vi "nanocal -- nuclear schottky fit V5.vi"() -> ()   [LabVIEW 2020]
uses:
  filename-pattern.ctl
  show-win- control.ctl
  cursor winow.ctl
  nanocal_data_read_format.ctl
  3-lorentzian-parameters.ctl
  nameformattingitem.ctl
  nanocal_side_selector.ctl
  filename-action.ctl
  nanocal -- gradient descent -- parameters.ctl
  3-lorentzian-heat-response action.ctl
  nanocal-goodness-weighting-strategy.ctl
  <vilib>/Analysis/Matrix/Datatypes/RealMatrix.ctl
  <vilib>/Analysis/Matrix/Datatypes/ComplexMatrix.ctl
  cursor window action.ctl
  cursor action.ctl
  2Dwindow.ctl
  publisher action.ctl
  <vilib>/Utility/miscctls.llb/LVMapReplaceAction.ctl
  mathematica string map action.ctl
  agregator -- action.ctl
  nanocal -- gradient descent -- action.ctl
  array action.ctl
  cursor sate.ctl
  nanocal -- defaut parameter manager action-- V1.ctl
  nanocal -- plotstring file action.ctl
  file -- read-write control.ctl
  array -- freq-voltage transformations action.ctl
  nanocal_raw_file_manage_action_V1.ctl
  KM_file -- read-write control.ctl
  replace cursor action stack.vi
  Q -- range multiplier -- real -- V2.vi
  Q - not nan and gtr than zero - Real.vi
  Q - not nan -- real.vi
  Q -- check range -- i -- real.vi
  array - smart min max.vi
  3-lorentzian-heat-response -- V4.vi/142dd4c5-f9ed-c64b-bc14-a88e3e2c450a.vi
  array -- freq-voltage transformations.vi/05c44075-957c-bc42-b6fa-2799d0bc0485.vi
  tale of three indices.vi
  filter -- window span logic.vi
  linear interp iiii- complex - z-omega - divide.vi
  linear interpolation iiii- complex.vi
  containing bix.vi
  <vilib>/Array/Sort 2D Array - Pop Stack.vi
  <vilib>/Array/Sort 2D Array - Push Stack.vi
  array -- freq-voltage transformations.vi/05c44075-957c-bc42-b6fa-2799d0bc0485.vi/5dd0d2be-718e-c148-b8fa-e083cdba2843.vi
  array -- freq-voltage transformations.vi/05c44075-957c-bc42-b6fa-2799d0bc0485.vi/095795a0-771d-c341-9fed-d90d2e44c51c.vi
  command stack.vi
  tale of three indices -- check state.vi
  Q -- check range -- i -- integer.vi
  linear interp iiii- complex - z-omega.vi
  line -- complex.vi
  Q - not nan -- integer.vi
  <vilib>/Analysis/baseanly.llb/A x B.vi
  <vilib>/Analysis/baseanly.llb/Complex A x B.vi
  <vilib>/Analysis/polynomials.llb/Polynomial Roots.vi
  <vilib>/Analysis/polynomials.llb/Polynomial Roots (DBL).vi
  <vilib>/Analysis/Matrix/Numeric/Conversions/Array To Matrix.vi
  <vilib>/Analysis/Matrix/Numeric/Conversions/Array To Matrix - RA2.vi
  <vilib>/Analysis/baseanly.llb/Inverse Matrix.vi
  <vilib>/Analysis/baseanly.llb/Real Inverse Matrix.vi
  <vilib>/Comparison/Less/Less Functor/Less Functor.lvclass
  <vilib>/Analysis/Matrix/NI_Matrix.lvlib
panel:
  in  "tab 10":enum32{"Page 1"}(tab)
  out "curvature tensor":T3
  in  "update curvature plots":bool
  in  "hist size":i32=300
  out "Plot: curvature":cluster{"Freq out (Hz)":dbl[], dbl[]}[](graph)=[{"Freq out (Hz)"=array[300 elements], array[300 elements]}, {"Freq out (Hz)"=[0.04153243950651924, 0.04180026172835088, 0.04258445003699314, 0.0438342337113713, 0.04546073322883233, 0.047333784316083864, 0.049283479875020374, 0.051110588081317194, 0.05260805187888057, 0.05359172755671921, 0.05393366537480654, 0.05358810212962696, 0.05260128268882461, 0.05110153651352443, 0.049273219665611157, 0.04732342294006821, 0.04545126886787391, 0.04382647076923001, 0.042578970605129884, 0.041797433982199705], [0.13184488900598287, 0.13171129861070444, 0.13163855142156844, 0.1316336653013922, 0.13169711120219474, 0.13182276985071803, 0.1319984960783584, 0.13220724864159986, 0.13242869729069096, 0.13264117301723377, 0.13282378589345417, 0.13295850464763131, 0.1330319812802772, 0.13303691930465214, 0.13297282794297968, 0.13284607301385357, 0.13266921842867932, 0.132459736424517, 0.13223823587146255, 0.13202640560334603]}]
  in  "scale gauge: Plot: curvatures":dbl(slide)=0.003141 min=0.0 max=0.3 step=1e-06 scale=1e-09..1.0 scale format="%#_3p"
  in  "radius factor":dbl(slide)=0.01 scale=0.001..1.0 scale format="%#_2p"
  in  "ellipse factor":dbl(slide)=0.0032728445121842026 scale=0.001..1.0 scale format="%#_2p"
  in  "tab 8":enum32{"main", "energy profile", "internals"}(tab)
  out "|dln G/dln α_i |":dbl(slide)=0.0009321298273703344 scale=1e-09..1.0 scale format="%#_3p"
  out "Goodness":dbl(slide)=0.04084184503494657 scale=0.0001..0.5 scale format="%#_3p"
  in  "sweeper panel":enum32{"main"}(tab)
  out "Plot: circles":cluster{"Freq out (Hz)":dbl[], dbl[]}[](graph)
  in  "scale gauge: Plot: circles":dbl(slide)=149590820.049497 min=0.0 max=0.3 step=1e-06 scale=10000000.0..10000000000.0 scale format="%#_3p"
  in  "cspan":dbl=0.003 format="%#_13g"
  in  "tab 77":enum32{"logarithmic derivatives"}(tab)
  in  "factors":cluster{"scaling":dbl, "what":T4}[](array[cluster])=[{"scaling"=1.0, "what"=enum."ζ"}, {"scaling"=1.0, "what"=enum."τ1"}, {"scaling"=1.0, "what"=enum."τS"}, {"scaling"=1.0, "what"=enum."τN"}, {"scaling"=1.0, "what"=enum."τC"}, {"scaling"=1.0, "what"=enum."κ0"}]
  in  "tab77":enum32{"Page 1"}(tab)
  in  "τC":dbl(slide)=0.0011273373743225924 min=0.0 max=0.3 step=1e-06 scale=0.0001..1.0 scale format="%#_3p"
  in  "τN":dbl(slide)=0.017465668384145063 min=0.0 max=0.3 step=1e-06 scale=1e-06..1.0 scale format="%#_3p"
  in  "τS":dbl(slide)=0.1325659964000386 min=0.0 max=0.3 step=1e-06 scale=0.0001..1.0 scale format="%#_3p"
  in  "ζ":dbl(slide)=0.29191584737823423 min=0.0 max=0.3 step=1e-06 scale=1e-05..1.0 scale format="%#_3p"
  in  "T1":dbl(slide)=0.04810958675443226 min=0.0 max=0.3 step=1e-06 scale=0.0001..1.0 scale format="%#_3p"
  in  "κ0":dbl(slide)=6.401292880383811e-10 min=0.0 max=0.3 step=1e-12 scale=1e-10..1e-06 scale format="%#_3p"
  in  "newton parameters":T5={"newton action"=enum."onlygrads", "weighting"=enum."dω √(|dz/dω|)", "PID-P"=0.00918775844298404, "PID-I"=5} {"PID-P" scale=1e-09..1.0 scale format="%#_3p"}
  out "vector v=dlogG/dlogα of logarithmic derivatives":dbl[](array[numeric])=[-3.065919719494306e-06, -0.0007578980980653129, -7.802452151739537e-05, 0.0005349845415649405, -7.224415710242577e-07, 2.2288197381997078e-07] format="%#11.9f"
  in  "tab 4":enum32{"Page 1"}(tab)
  in  "go / pause!":bool
  in  "plots tab":enum32{"Page 1"}(tab)
  in  "X selector":T4=enum."T (K)"
  out "Plot:  colors":cluster{"Freq out (Hz)":dbl[], dbl[]}[](graph)=[{"Freq out (Hz)"=[0.122, 0.157, 0.17, 0.197, 0.255, 0.308, 0.36, 0.438, 0.53, 0.62], [0.39349272631, 0.29106997063, 0.268635074603, 0.206153415117, 0.118203366926, 0.082420645473, 0.059658452725, 0.044694234886, 0.035816355504, 0.030262302634]}, {"Freq out (Hz)"=[0.122, 0.157, 0.17, 0.197, 0.255, 0.308, 0.36, 0.438, 0.53, 0.62], [0.051042943794, 0.041769159443, 0.043057144668, 0.034947930436, 0.027744681967, 0.02481742265, 0.023285662985, 0.019992829849, 0.018852618665, 0.017398280529]}, {"Freq out (Hz)"=[0.122, 0.157, 0.17, 0.197, 0.255, 0.308, 0.36, 0.438, 0.53, 0.62], [0.190886011231, 0.12886574092, 0.111204314939, 0.084522761663, 0.059746199179, 0.049602237526, 0.042805762544, 0.035923567004, 0.030539930714, 0.027078056707]}, {"Freq out (Hz)"=[0.122, 0.157, 0.17, 0.197, 0.255, 0.308, 0.36, 0.438, 0.53, 0.62], [0.068025612152, 0.021652136843, 0.015435608341, 0.010857436832, 0.005820820615, 0.002810348987, 0.001792307846, 0.001180276169, 0.000576682499, 0.000382363637]}, {"Freq out (Hz)"=[0.122, 0.157, 0.17, 0.197, 0.255, 0.308, 0.36, 0.438, 0.53, 0.62], [0.00123122126, 0.001128336098, 0.001079948561, 0.00111922842, 0.001318444261, 0.001541254413, 0.001977636623, 0.002238202456, 0.002754969701, 0.002680781698]}]
  in  "tab 55":T8(tab)=enum."oscillations"
  in  "string IN":string="  \"IDS0158_210310_RAW_cal__ref_\" ->   <|    \"ζ\" -> 0.331549170129   ,  \"τ1\" -> 0.031957261989   ,  \"τS\" -> 0.245155954508   ,  \"τN\" -> 0.327332604975   ,  \"τC\" -> 0.001044440547   ,  \"κ0\" -> 0.000000000511   ,  \"mm1\" -> 0.000259429775   ,  \"mm2\" -> 0.013378446840   ,  \"mm3\" -> 0.781660492209   ,  \"T\" -> 0.140000000000   ,  \"B\" -> 12.000000000000   ,  \"θ\" -> 0.000000000000   ,  \"Reoff\" -> 0.000000000000   ,  \"Imoff\" -> 0.000000000000    |>   , \r\"IDS0158_210310_RAW_cal__sam_\" ->   <|    \"ζ\" -> 0.286336668596   ,  \"τ1\" -> 0.037477267671   ,  \"τS\" -> 0.354459287884   ,  \"τN\" -> 0.444916383639   ,  \"τC\" -> 0.001225600579   ,  \"κ0\" -> 0.000000000596   ,  \"mm1\" -> 0.000272242393   ,  \"mm2\" -> 0.016302418461   ,  \"mm3\" -> 1.050394445660   ,  \"T\" -> 0.140000000000   ,  \"B\" -> 12.000000000000   ,  \"θ\" -> 0.000000000000   ,  \"Reoff\" -> 0.000000000000   ,  \"Imoff\" -> 0.000000000000    |>   , \r\"IDS0159_210310_RAW_cal__ref_\" ->   <|    \"ζ\" -> 0.269623663752   ,  \"τ1\" -> 0.029946823009   ,  \"τS\" -> 0.193020268264   ,  \"τN\" -> 0.181925572107   ,  \"τC\" -> 0.001029221853   ,  \"κ0\" -> 0.000000000645   ,  \"mm1\" -> 0.000217844451   ,  \"mm2\" -> 0.014971381157   ,  \"mm3\" -> 0.491826930814   ,  \"T\" -> 0.170000000000   ,  \"B\" -> 12.000000000000   ,  \"θ\" -> 0.000000000000   ,  \"Reoff\" -> 0.000000000000   ,  \"Imoff\" -> 0.000000000000    |>   , \r\"IDS0159_210310_RAW_cal__sam_\" ->   <|    \"ζ\" -> 0.219100303741   ,  \"τ1\" -> 0.028643012604   ,  \"τS\" -> 0.279362928811   ,  \"τN\" -> 0.246156444058   ,  \"τC\" -> 0.001272401549   ,  \"κ0\" -> 0.000000000760   ,  \"mm1\" -> 0.000227975653   ,  \"mm2\" -> 0.014929571562   ,  \"mm3\" -> 0.655418694024   ,  \"T\" -> 0.170000000000   ,  \"B\" -> 12.000000000000   ,  \"θ\" -> 0.000000000000   ,  \"Reoff\" -> 0.000000000000   ,  \"Imoff\" -> 0.000000000000    |>   , \r\"IDS0160_210310_RAW_cal__ref_\" ->   <|    \"ζ\" -> 0.207047266456   ,  \"τ1\" -> 0.027475093360   ,  \"τS\" -> 0.117497913331   ,  \"τN\" -> 0.102020652890   ,  \"τC\" -> 0.000950950989   ,  \"κ0\" -> 0.000000000918   ,  \"mm1\" -> 0.000162211763   ,  \"mm2\" -> 0.014034650200   ,  \"mm3\" -> 0.279198467680   ,  \"T\" -> 0.200000000000   ,  \"B\" -> 12.000000000000   ,  \"θ\" -> 0.000000000000   ,  \"Reoff\" -> 0.000000000000   ,  \"Imoff\" -> 0.000000000000    |>   , \r\"IDS0160_210310_RAW_cal__sam_\" ->   <|    \"ζ\" -> 0.170488637524   ,  \"τ1\" -> 0.029234231120   ,  \"τS\" -> 0.149095458227   ,  \"τN\" -> 0.151792620275   ,  \"τC\" -> 0.001113424175   ,  \"κ0\" -> 0.000000001042   ,  \"mm1\" -> 0.000161291869   ,  \"mm2\" -> 0.013922632736   ,  \"mm3\" -> 0.368449807743   ,  \"T\" -> 0.200000000000   ,  \"B\" -> 12.000000000000   ,  \"θ\" -> 0.000000000000   ,  \"Reoff\" -> 0.000000000000   ,  \"Imoff\" -> 0.000000000000    |>   , \r\"IDS0161_210310_RAW_cal__ref_\" ->   <|    \"ζ\" -> 0.165418845287   ,  \"τ1\" -> 0.025256902580   ,  \"τS\" -> 0.095232124148   ,  \"τN\" -> 0.068477414693   ,  \"τC\" -> 0.001100413424   ,  \"κ0\" -> 0.000000001058   ,  \"mm1\" -> 0.000154866739   ,  \"mm2\" -> 0.013921914824   ,  \"mm3\" -> 0.203070716160   ,  \"T\" -> 0.220000000000   ,  \"B\" -> 12.000000000000   ,  \"θ\" -> 0.000000000000   ,  \"Reoff\" -> 0.000000000000   ,  \"Imoff\" -> 0.000000000000    |>   , \r\"IDS0161_210310_RAW_cal__sam_\" ->   <|    \"ζ\" -> 0.130531197151   ,  \"τ1\" -> 0.025704482770   ,  \"τS\" -> 0.129606657196   ,  \"τN\" -> 0.091602369165   ,  \"τC\" -> 0.001441379995   ,  \"κ0\" -> 0.000000001211   ,  \"mm1\" -> 0.000164978070   ,  \"mm2\" -> 0.014468182937   ,  \"mm3\" -> 0.262596407151   ,  \"T\" -> 0.220000000000   ,  \"B\" -> 12.000000000000   ,  \"θ\" -> 0.000000000000   ,  \"Reoff\" -> 0.000000000000   ,  \"Imoff\" -> 0.000000000000    |>   , \r\"IDS0162_210310_RAW_cal__ref_\" ->   <|    \"ζ\" -> 0.094488415983   ,  \"τ1\" -> 0.023440091411   ,  \"τS\" -> 0.070629137621   ,  \"τN\" -> 0.023695223047   ,  \"τC\" -> 0.001462465509   ,  \"κ0\" -> 0.000000001371   ,  \"mm1\" -> 0.000124103809   ,  \"mm2\" -> 0.016535879819   ,  \"mm3\" -> 0.111479493388   ,  \"T\" -> 0.280000000000   ,  \"B\" -> 12.000000000000   ,  \"θ\" -> 0.000000000000   ,  \"Reoff\" -> 0.000000000000   ,  \"Imoff\" -> 0.000000000000    |>   , \r\"IDS0162_210310_RAW_cal__sam_\" ->   <|    \"ζ\" -> 0.078258046754   ,  \"τ1\" -> 0.028009840731   ,  \"τS\" -> 0.092122038762   ,  \"τN\" -> 0.030129595899   ,  \"τC\" -> 0.001641062244   ,  \"κ0\" -> 0.000000001543   ,  \"mm1\" -> 0.000117303440   ,  \"mm2\" -> 0.019983073008   ,  \"mm3\" -> 0.141369335330   ,  \"T\" -> 0.280000000000   ,  \"B\" -> 12.000000000000   ,  \"θ\" -> 0.000000000000   ,  \"Reoff\" -> 0.000000000000   ,  \"Imoff\" -> 0.000000000000    |>   , \r\"IDS0163_210310_RAW_cal__ref_\" ->   <|    \"ζ\" -> 0.066045279838   ,  \"τ1\" -> 0.021690723483   ,  \"τS\" -> 0.054398710223   ,  \"τN\" -> 0.012159058060   ,  \"τC\" -> 0.001677829713   ,  \"κ0\" -> 0.000000001745   ,  \"mm1\" -> 0.000101193423   ,  \"mm2\" -> 0.016659114676   ,  \"mm3\" -> 0.077561839811   ,  \"T\" -> 0.330000000000   ,  \"B\" -> 12.000000000000   ,  \"θ\" -> 0.000000000000   ,  \"Reoff\" -> 0.000000000000   ,  \"Imoff\" -> 0.000000000000    |>   , \r\"IDS0163_210310_RAW_cal__sam_\" ->   <|    \"ζ\" -> 0.054088186012   ,  \"τ1\" -> 0.023838802615   ,  \"τS\" -> 0.069079396629   ,  \"τN\" -> 0.016435267456   ,  \"τC\" -> 0.002025071743   ,  \"κ0\" -> 0.000000001955   ,  \"mm1\" -> 0.000101234646   ,  \"mm2\" -> 0.018244822177   ,  \"mm3\" -> 0.097657814678   ,  \"T\" -> 0.330000000000   ,  \"B\" -> 12.000000000000   ,  \"θ\" -> 0.000000000000   ,  \"Reoff\" -> 0.000000000000   ,  \"Imoff\" -> 0.000000000000    |>   , \r\"IDS0164_210310_RAW_cal__ref_\" ->   <|    \"ζ\" -> 0.046429657722   ,  \"τ1\" -> 0.021005913305   ,  \"τS\" -> 0.044250298502   ,  \"τN\" -> 0.006399419767   ,  \"τC\" -> 0.002349605146   ,  \"κ0\" -> 0.000000002166   ,  \"mm1\" -> 0.000099416540   ,  \"mm2\" -> 0.017300257108   ,  \"mm3\" -> 0.058957212156   ,  \"T\" -> 0.400000000000   ,  \"B\" -> 12.000000000000   ,  \"θ\" -> 0.000000000000   ,  \"Reoff\" -> 0.000000000000   ,  \"Imoff\" -> 0.000000000000    |>   , \r\"IDS0164_210310_RAW_cal__sam_\" ->   <|    \"ζ\" -> 0.039314966212   ,  \"τ1\" -> 0.020712803909   ,  \"τS\" -> 0.055413767550   ,  \"τN\" -> 0.008474403424   ,  \"τC\" -> 0.002674063387   ,  \"κ0\" -> 0.000000002415   ,  \"mm1\" -> 0.000096818147   ,  \"mm2\" -> 0.017190811405   ,  \"mm3\" -> 0.072499170001   ,  \"T\" -> 0.400000000000   ,  \"B\" -> 12.000000000000   ,  \"θ\" -> 0.000000000000   ,  \"Reoff\" -> 0.000000000000   ,  \"Imoff\" -> 0.000000000000    |>   , \r\"IDS0165_210310_RAW_cal__ref_\" ->   <|    \"ζ\" -> 0.033449822896   ,  \"τ1\" -> 0.018946770596   ,  \"τS\" -> 0.035864277160   ,  \"τN\" -> 0.004007639534   ,  \"τC\" -> 0.003128970761   ,  \"κ0\" -> 0.000000002686   ,  \"mm1\" -> 0.000093605726   ,  \"mm2\" -> 0.016154023077   ,  \"mm3\" -> 0.047033737800   ,  \"T\" -> 0.480000000000   ,  \"B\" -> 12.000000000000   ,  \"θ\" -> 0.000000000000   ,  \"Reoff\" -> 0.000000000000   ,  \"Imoff\" -> 0.000000000000    |>   , \r\"IDS0165_210310_RAW_cal__sam_\" ->   <|    \"ζ\" -> 0.031945976845   ,  \"τ1\" -> 0.019000922826   ,  \"τS\" -> 0.045624146388   ,  \"τN\" -> 0.005314716063   ,  \"τC\" -> 0.002488383471   ,  \"κ0\" -> 0.000000002954   ,  \"mm1\" -> 0.000073272643   ,  \"mm2\" -> 0.016306894362   ,  \"mm3\" -> 0.057675293464   ,  \"T\" -> 0.480000000000   ,  \"B\" -> 12.000000000000   ,  \"θ\" -> 0.000000000000   ,  \"Reoff\" -> 0.000000000000   ,  \"Imoff\" -> 0.000000000000    |>   , \r\"IDS0166_210310_RAW_cal__ref_\" ->   <|    \"ζ\" -> 0.026131121682   ,  \"τ1\" -> 0.018837612836   ,  \"τS\" -> 0.029051745056   ,  \"τN\" -> 0.002477027845   ,  \"τC\" -> 0.003638595201   ,  \"κ0\" -> 0.000000003369   ,  \"mm1\" -> 0.000082781476   ,  \"mm2\" -> 0.016386279858   ,  \"mm3\" -> 0.038359801806   ,  \"T\" -> 0.580000000000   ,  \"B\" -> 12.000000000000   ,  \"θ\" -> 0.000000000000   ,  \"Reoff\" -> 0.000000000000   ,  \"Imoff\" -> 0.000000000000    |>   , \r\"IDS0166_210310_RAW_cal__sam_\" ->   <|    \"ζ\" -> 0.023031239946   ,  \"τ1\" -> 0.018268814012   ,  \"τS\" -> 0.037269400776   ,  \"τN\" -> 0.002696792890   ,  \"τC\" -> 0.003257395394   ,  \"κ0\" -> 0.000000003720   ,  \"mm1\" -> 0.000067670174   ,  \"mm2\" -> 0.016445281937   ,  \"mm3\" -> 0.045899921957   ,  \"T\" -> 0.580000000000   ,  \"B\" -> 12.000000000000   ,  \"θ\" -> 0.000000000000   ,  \"Reoff\" -> 0.000000000000   ,  \"Imoff\" -> 0.000000000000    |>   , \r\"IDS0167_210310_RAW_cal__ref_\" ->   <|    \"ζ\" -> 0.026557278794   ,  \"τ1\" -> 0.016933945977   ,  \"τS\" -> 0.022881111855   ,  \"τN\" -> 0.001392473895   ,  \"τC\" -> 0.004119437148   ,  \"κ0\" -> 0.000000003981   ,  \"mm1\" -> 0.000090964667   ,  \"mm2\" -> 0.015177563241   ,  \"mm3\" -> 0.030703081351   ,  \"T\" -> 0.680000000000   ,  \"B\" -> 12.000000000000   ,  \"θ\" -> 0.000000000000   ,  \"Reoff\" -> 0.000000000000   ,  \"Imoff\" -> 0.000000000000    |>   , \r\"IDS0167_210310_RAW_cal__sam_\" ->   <|    \"ζ\" -> 0.019920170845   ,  \"τ1\" -> 0.016368892412   ,  \"τS\" -> 0.030579536580   ,  \"τN\" -> 0.001736017565   ,  \"τC\" -> 0.004971418152   ,  \"κ0\" -> 0.000000004410   ,  \"mm1\" -> 0.000083939556   ,  \"mm2\" -> 0.015095997595   ,  \"mm3\" -> 0.039119658918   ,  \"T\" -> 0.680000000000   ,  \"B\" -> 12.000000000000   ,  \"θ\" -> 0.000000000000   ,  \"Reoff\" -> 0.000000000000   ,  \"Imoff\" -> 0.000000000000    |>   , \r\"IDS0168_210310_RAW_cal__ref_\" ->   <|    \"ζ\" -> 0.022041296958   ,  \"τ1\" -> 0.014045615335   ,  \"τS\" -> 0.018889590451   ,  \"τN\" -> 0.000813465770   ,  \"τC\" -> 0.004122617309   ,  \"κ0\" -> 0.000000005540   ,  \"mm1\" -> 0.000073491061   ,  \"mm2\" -> 0.013002629707   ,  \"mm3\" -> 0.025229449010   ,  \"T\" -> 0.910000000000   ,  \"B\" -> 12.000000000000   ,  \"θ\" -> 0.000000000000   ,  \"Reoff\" -> 0.000000000000   ,  \"Imoff\" -> 0.000000000000    |>   , \r\"IDS0168_210310_RAW_cal__sam_\" ->   <|    \"ζ\" -> 0.017558473054   ,  \"τ1\" -> 0.014545104284   ,  \"τS\" -> 0.022979681288   ,  \"τN\" -> 0.000840829385   ,  \"τC\" -> 0.005228030240   ,  \"κ0\" -> 0.000000006068   ,  \"mm1\" -> 0.000073916527   ,  \"mm2\" -> 0.013750428362   ,  \"mm3\" -> 0.030187552103   ,  \"T\" -> 0.910000000000   ,  \"B\" -> 12.000000000000   ,  \"θ\" -> 0.000000000000   ,  \"Reoff\" -> 0.000000000000   ,  \"Imoff\" -> 0.000000000000    |>   , \r\"IDS0169_210310_RAW_cal__ref_\" ->   <|    \"ζ\" -> 0.021090283514   ,  \"τ1\" -> 0.013945744068   ,  \"τS\" -> 0.014386606899   ,  \"τN\" -> 0.000345175874   ,  \"τC\" -> 0.004902956629   ,  \"κ0\" -> 0.000000007742   ,  \"mm1\" -> 0.000076221408   ,  \"mm2\" -> 0.013209066715   ,  \"mm3\" -> 0.020605892822   ,  \"T\" -> 1.230000000000   ,  \"B\" -> 12.000000000000   ,  \"θ\" -> 0.000000000000   ,  \"Reoff\" -> 0.000000000000   ,  \"Imoff\" -> 0.000000000000    |>   , \r\"IDS0169_210310_RAW_cal__sam_\" ->   <|    \"ζ\" -> 0.011916480594   ,  \"τ1\" -> 0.012551282481   ,  \"τS\" -> 0.018233218660   ,  \"τN\" -> 0.000345702746   ,  \"τC\" -> 0.004699451527   ,  \"κ0\" -> 0.000000008451   ,  \"mm1\" -> 0.000044190864   ,  \"mm2\" -> 0.012162820727   ,  \"mm3\" -> 0.023844039179   ,  \"T\" -> 1.230000000000   ,  \"B\" -> 12.000000000000   ,  \"θ\" -> 0.000000000000   ,  \"Reoff\" -> 0.000000000000   ,  \"Imoff\" -> 0.000000000000    |>   , \r\"IDS0170_210310_RAW_cal__ref_\" ->   <|    \"ζ\" -> 0.021449250230   ,  \"τ1\" -> 0.014564522147   ,  \"τS\" -> 0.008878867204   ,  \"τN\" -> 0.000064984242   ,  \"τC\" -> 0.006207353748   ,  \"κ0\" -> 0.000000012530   ,  \"mm1\" -> 0.000077778127   ,  \"mm2\" -> 0.013872772336   ,  \"mm3\" -> 0.015957015786   ,  \"T\" -> 1.970000000000   ,  \"B\" -> 12.000000000000   ,  \"θ\" -> 0.000000000000   ,  \"Reoff\" -> 0.000000000000   ,  \"Imoff\" -> 0.000000000000    |>   , \r\"IDS0170_210310_RAW_cal__sam_\" ->   <|    \"ζ\" -> 0.012831327568   ,  \"τ1\" -> 0.013315909415   ,  \"τS\" -> 0.012590836847   ,  \"τN\" -> 0.000065003013   ,  \"τC\" -> 0.005276356243   ,  \"κ0\" -> 0.000000013610   ,  \"mm1\" -> 0.000047406274   ,  \"mm2\" -> 0.013137605540   ,  \"mm3\" -> 0.018225484932   ,  \"T\" -> 1.970000000000   ,  \"B\" -> 12.000000000000   ,  \"θ\" -> 0.000000000000   ,  \"Reoff\" -> 0.000000000000   ,  \"Imoff\" -> 0.000000000000    |>   , \r\"IDS0171_210310_RAW_cal__ref_\" ->   <|    \"ζ\" -> 0.024633693577   ,  \"τ1\" -> 0.014940694735   ,  \"τS\" -> 0.006137734482   ,  \"τN\" -> 0.000014567254   ,  \"τC\" -> 0.005080683927   ,  \"κ0\" -> 0.000000022488   ,  \"mm1\" -> 0.000067969819   ,  \"mm2\" -> 0.011256263587   ,  \"mm3\" -> 0.015001000908   ,  \"T\" -> 3.190000000000   ,  \"B\" -> 12.000000000000   ,  \"θ\" -> 0.000000000000   ,  \"Reoff\" -> 0.000000000000   ,  \"Imoff\" -> 0.000000000000    |>   , \r\"IDS0171_210310_RAW_cal__sam_\" ->   <|    \"ζ\" -> 0.019774146838   ,  \"τ1\" -> 0.013257273421   ,  \"τS\" -> 0.007064131508   ,  \"τN\" -> 0.000028000819   ,  \"τC\" -> 0.006942241845   ,  \"κ0\" -> 0.000000023477   ,  \"mm1\" -> 0.000068886863   ,  \"mm2\" -> 0.012935419574   ,  \"mm3\" -> 0.014427582022   ,  \"T\" -> 3.190000000000   ,  \"B\" -> 12.000000000000   ,  \"θ\" -> 0.000000000000   ,  \"Reoff\" -> 0.000000000000   ,  \"Imoff\" -> 0.000000000000    |>   , \r\"IDS0172_210310_RAW_cal__ref_\" ->   <|    \"ζ\" -> 0.027835388666   ,  \"τ1\" -> 0.013976390421   ,  \"τS\" -> 0.003539188638   ,  \"τN\" -> 0.000003774856   ,  \"τC\" -> 0.004420299329   ,  \"κ0\" -> 0.000000055482   ,  \"mm1\" -> 0.000054408485   ,  \"mm2\" -> 0.007998445403   ,  \"mm3\" -> 0.013985419121   ,  \"T\" -> 5.800000000000   ,  \"B\" -> 12.000000000000   ,  \"θ\" -> 0.000000000000   ,  \"Reoff\" -> 0.000000000000   ,  \"Imoff\" -> 0.000000000000    |>   , \r\"IDS0172_210310_RAW_cal__sam_\" ->   <|    \"ζ\" -> 0.029251354442   ,  \"τ1\" -> 0.014634751206   ,  \"τS\" -> 0.003873958746   ,  \"τN\" -> 0.000007000487   ,  \"τC\" -> 0.006827504775   ,  \"κ0\" -> 0.000000056438   ,  \"mm1\" -> 0.000072018576   ,  \"mm2\" -> 0.010723236476   ,  \"mm3\" -> 0.014661483476   ,  \"T\" -> 5.800000000000   ,  \"B\" -> 12.000000000000   ,  \"θ\" -> 0.000000000000   ,  \"Reoff\" -> 0.000000000000   ,  \"Imoff\" -> 0.000000000000    |>   , \r\"IDS0181_210310_RAW_cal__ref_\" ->   <|    \"ζ\" -> 0.194847779603   ,  \"τ1\" -> 0.071300022200   ,  \"τS\" -> 0.034370433557   ,  \"τN\" -> 0.119698958932   ,  \"τC\" -> 0.001245041457   ,  \"κ0\" -> 0.000000000909   ,  \"mm1\" -> 0.000197936786   ,  \"mm2\" -> 0.012302667617   ,  \"mm3\" -> 0.244133930774   ,  \"T\" -> 0.179000000000   ,  \"B\" -> 12.000000000000   ,  \"θ\" -> 90.000000000000   ,  \"Reoff\" -> 0.000000000000   ,  \"Imoff\" -> 0.000000000000    |>   , \r\"IDS0181_210310_RAW_cal__sam_\" ->   <|    \"ζ\" -> 0.161975781729   ,  \"τ1\" -> 0.073089805113   ,  \"τS\" -> 0.045018408115   ,  \"τN\" -> 0.161987434028   ,  \"τC\" -> 0.001482104484   ,  \"κ0\" -> 0.000000001038   ,  \"mm1\" -> 0.000201615809   ,  \"mm2\" -> 0.012976126678   ,  \"mm3\" -> 0.301929942357   ,  \"T\" -> 0.179000000000   ,  \"B\" -> 12.000000000000   ,  \"θ\" -> 90.000000000000   ,  \"Reoff\" -> 0.000000000000   ,  \"Imoff\" -> 0.000000000000    |>   , \r\"IDS0183_210310_RAW_cal__ref_\" ->   <|    \"ζ\" -> 0.368639553991   ,  \"τ1\" -> 0.116941860160   ,  \"τS\" -> 0.051705641175   ,  \"τN\" -> 0.670097053448   ,  \"τC\" -> 0.001215131262   ,  \"κ0\" -> 0.000000000441   ,  \"mm1\" -> 0.000323068314   ,  \"mm2\" -> 0.007634876736   ,  \"mm3\" -> 1.098086764410   ,  \"T\" -> 0.120000000000   ,  \"B\" -> 12.000000000000   ,  \"θ\" -> 90.000000000000   ,  \"Reoff\" -> 0.000000000000   ,  \"Imoff\" -> 0.000000000000    |>   , \r\"IDS0183_210310_RAW_cal__sam_\" ->   <|    \"ζ\" -> 0.300863384227   ,  \"τ1\" -> 0.104924004009   ,  \"τS\" -> 0.071070599729   ,  \"τN\" -> 0.992887187112   ,  \"τC\" -> 0.001721587800   ,  \"κ0\" -> 0.000000000548   ,  \"mm1\" -> 0.000392216822   ,  \"mm2\" -> 0.006637384427   ,  \"mm3\" -> 1.483679717825   ,  \"T\" -> 0.120000000000   ,  \"B\" -> 12.000000000000   ,  \"θ\" -> 90.000000000000   ,  \"Reoff\" -> 0.000000000000   ,  \"Imoff\" -> 0.000000000000    |>   , \r\"IDS0184_210310_RAW_cal__ref_\" ->   <|    \"ζ\" -> 0.260731272629   ,  \"τ1\" -> 0.088447317905   ,  \"τS\" -> 0.043671964304   ,  \"τN\" -> 0.254005375090   ,  \"τC\" -> 0.001151280234   ,  \"κ0\" -> 0.000000000662   ,  \"mm1\" -> 0.000234134476   ,  \"mm2\" -> 0.010914094163   ,  \"mm3\" -> 0.453741500427   ,  \"T\" -> 0.148000000000   ,  \"B\" -> 12.000000000000   ,  \"θ\" -> 90.000000000000   ,  \"Reoff\" -> 0.000000000000   ,  \"Imoff\" -> 0.000000000000    |>   , \r\"IDS0184_210310_RAW_cal__sam_\" ->   <|    \"ζ\" -> 0.215697702358   ,  \"τ1\" -> 0.095971807771   ,  \"τS\" -> 0.069319630290   ,  \"τN\" -> 0.366712218878   ,  \"τC\" -> 0.001526252261   ,  \"κ0\" -> 0.000000000784   ,  \"mm1\" -> 0.000266752031   ,  \"mm2\" -> 0.013373263674   ,  \"mm3\" -> 0.613940961515   ,  \"T\" -> 0.148000000000   ,  \"B\" -> 12.000000000000   ,  \"θ\" -> 90.000000000000   ,  \"Reoff\" -> 0.000000000000   ,  \"Imoff\" -> 0.000000000000    |>   , \r\"IDS0185_210310_RAW_cal__ref_\" ->   <|    \"ζ\" -> 0.166318035375   ,  \"τ1\" -> 0.066119695107   ,  \"τS\" -> 0.031891479777   ,  \"τN\" -> 0.088107606578   ,  \"τC\" -> 0.001299933301   ,  \"κ0\" -> 0.000000001075   ,  \"mm1\" -> 0.000179913074   ,  \"mm2\" -> 0.013052011118   ,  \"mm3\" -> 0.194144802860   ,  \"T\" -> 0.197000000000   ,  \"B\" -> 12.000000000000   ,  \"θ\" -> 90.000000000000   ,  \"Reoff\" -> 0.000000000000   ,  \"Imoff\" -> 0.000000000000    |>   , \r\"IDS0185_210310_RAW_cal__sam_\" ->   <|    \"ζ\" -> 0.139117463690   ,  \"τ1\" -> 0.070330410174   ,  \"τS\" -> 0.040829719954   ,  \"τN\" -> 0.122434321115   ,  \"τC\" -> 0.001436112939   ,  \"κ0\" -> 0.000000001208   ,  \"mm1\" -> 0.000170710071   ,  \"mm2\" -> 0.013785404893   ,  \"mm3\" -> 0.243787328523   ,  \"T\" -> 0.197000000000   ,  \"B\" -> 12.000000000000   ,  \"θ\" -> 90.000000000000   ,  \"Reoff\" -> 0.000000000000   ,  \"Imoff\" -> 0.000000000000    |>   , \r\"IDS0186_210310_RAW_cal__ref_\" ->   <|    \"ζ\" -> 0.101265410351   ,  \"τ1\" -> 0.051590946451   ,  \"τS\" -> 0.026920044229   ,  \"τN\" -> 0.035536954174   ,  \"τC\" -> 0.001490330879   ,  \"κ0\" -> 0.000000001364   ,  \"mm1\" -> 0.000131013977   ,  \"mm2\" -> 0.014987531242   ,  \"mm3\" -> 0.106744464087   ,  \"T\" -> 0.249000000000   ,  \"B\" -> 12.000000000000   ,  \"θ\" -> 90.000000000000   ,  \"Reoff\" -> 0.000000000000   ,  \"Imoff\" -> 0.000000000000    |>   , \r\"IDS0186_210310_RAW_cal__sam_\" ->   <|    \"ζ\" -> 0.079912790251   ,  \"τ1\" -> 0.053932962768   ,  \"τS\" -> 0.033847624645   ,  \"τN\" -> 0.047947649984   ,  \"τC\" -> 0.001828917906   ,  \"κ0\" -> 0.000000001546   ,  \"mm1\" -> 0.000129305669   ,  \"mm2\" -> 0.016142481427   ,  \"mm3\" -> 0.127821856832   ,  \"T\" -> 0.249000000000   ,  \"B\" -> 12.000000000000   ,  \"θ\" -> 90.000000000000   ,  \"Reoff\" -> 0.000000000000   ,  \"Imoff\" -> 0.000000000000    |>   , \r\"IDS0187_210310_RAW_cal__ref_\" ->   <|    \"ζ\" -> 0.070401604603   ,  \"τ1\" -> 0.043684283216   ,  \"τS\" -> 0.023756676354   ,  \"τN\" -> 0.017570167589   ,  \"τC\" -> 0.001809460237   ,  \"κ0\" -> 0.000000001742   ,  \"mm1\" -> 0.000111548159   ,  \"mm2\" -> 0.016126491037   ,  \"mm3\" -> 0.073492024327   ,  \"T\" -> 0.300000000000   ,  \"B\" -> 12.000000000000   ,  \"θ\" -> 90.000000000000   ,  \"Reoff\" -> 0.000000000000   ,  \"Imoff\" -> 0.000000000000    |>   , \r\"IDS0187_210310_RAW_cal__sam_\" ->   <|    \"ζ\" -> 0.057938569833   ,  \"τ1\" -> 0.045244527663   ,  \"τS\" -> 0.029709028064   ,  \"τN\" -> 0.023577376257   ,  \"τC\" -> 0.002006607539   ,  \"κ0\" -> 0.000000001948   ,  \"mm1\" -> 0.000103608352   ,  \"mm2\" -> 0.017542867394   ,  \"mm3\" -> 0.085978401835   ,  \"T\" -> 0.300000000000   ,  \"B\" -> 12.000000000000   ,  \"θ\" -> 90.000000000000   ,  \"Reoff\" -> 0.000000000000   ,  \"Imoff\" -> 0.000000000000    |>   , \r\"IDS0188_210310_RAW_cal__ref_\" ->   <|    \"ζ\" -> 0.052039078112   ,  \"τ1\" -> 0.037833987996   ,  \"τS\" -> 0.021664376950   ,  \"τN\" -> 0.010364100672   ,  \"τC\" -> 0.002302914949   ,  \"κ0\" -> 0.000000002119   ,  \"mm1\" -> 0.000103877861   ,  \"mm2\" -> 0.016533069886   ,  \"mm3\" -> 0.057195165269   ,  \"T\" -> 0.360000000000   ,  \"B\" -> 12.000000000000   ,  \"θ\" -> 90.000000000000   ,  \"Reoff\" -> 0.000000000000   ,  \"Imoff\" -> 0.000000000000    |>   , \r\"IDS0188_210310_RAW_cal__sam_\" ->   <|    \"ζ\" -> 0.044154556051   ,  \"τ1\" -> 0.038823125235   ,  \"τS\" -> 0.027069314930   ,  \"τN\" -> 0.013601990730   ,  \"τC\" -> 0.002287979276   ,  \"κ0\" -> 0.000000002359   ,  \"mm1\" -> 0.000089763345   ,  \"mm2\" -> 0.018083678254   ,  \"mm3\" -> 0.065404792018   ,  \"T\" -> 0.360000000000   ,  \"B\" -> 12.000000000000   ,  \"θ\" -> 90.000000000000   ,  \"Reoff\" -> 0.000000000000   ,  \"Imoff\" -> 0.000000000000    |>   , \r\"IDS0189_210310_RAW_cal__ref_\" ->   <|    \"ζ\" -> 0.040584680050   ,  \"τ1\" -> 0.030359591877   ,  \"τS\" -> 0.019792901852   ,  \"τN\" -> 0.005324821183   ,  \"τC\" -> 0.002700986774   ,  \"κ0\" -> 0.000000002671   ,  \"mm1\" -> 0.000093496766   ,  \"mm2\" -> 0.016559544569   ,  \"mm3\" -> 0.042544655105   ,  \"T\" -> 0.430000000000   ,  \"B\" -> 12.000000000000   ,  \"θ\" -> 90.000000000000   ,  \"Reoff\" -> 0.000000000000   ,  \"Imoff\" -> 0.000000000000    |>   , \r\"IDS0189_210310_RAW_cal__sam_\" ->   <|    \"ζ\" -> 0.032748569996   ,  \"τ1\" -> 0.031072007290   ,  \"τS\" -> 0.024343937548   ,  \"τN\" -> 0.006961654481   ,  \"τC\" -> 0.002967111565   ,  \"κ0\" -> 0.000000002964   ,  \"mm1\" -> 0.000084402249   ,  \"mm2\" -> 0.018055855929   ,  \"mm3\" -> 0.048229666078   ,  \"T\" -> 0.430000000000   ,  \"B\" -> 12.000000000000   ,  \"θ\" -> 90.000000000000   ,  \"Reoff\" -> 0.000000000000   ,  \"Imoff\" -> 0.000000000000    |>   , \r\"IDS0190_210310_RAW_cal__ref_\" ->   <|    \"ζ\" -> 0.030700897923   ,  \"τ1\" -> 0.026935085078   ,  \"τS\" -> 0.018364864329   ,  \"τN\" -> 0.002898516959   ,  \"τC\" -> 0.003150649099   ,  \"κ0\" -> 0.000000003342   ,  \"mm1\" -> 0.000080744936   ,  \"mm2\" -> 0.016939553323   ,  \"mm3\" -> 0.034981622105   ,  \"T\" -> 0.512000000000   ,  \"B\" -> 12.000000000000   ,  \"θ\" -> 90.000000000000   ,  \"Reoff\" -> 0.000000000000   ,  \"Imoff\" -> 0.000000000000    |>   , \r\"IDS0190_210310_RAW_cal__sam_\" ->   <|    \"ζ\" -> 0.027599263457   ,  \"τ1\" -> 0.026239105728   ,  \"τS\" -> 0.022370859308   ,  \"τN\" -> 0.003857632966   ,  \"τC\" -> 0.003499360499   ,  \"κ0\" -> 0.000000003681   ,  \"mm1\" -> 0.000081816106   ,  \"mm2\" -> 0.017901054668   ,  \"mm3\" -> 0.038707974796   ,  \"T\" -> 0.512000000000   ,  \"B\" -> 12.000000000000   ,  \"θ\" -> 90.000000000000   ,  \"Reoff\" -> 0.000000000000   ,  \"Imoff\" -> 0.000000000000    |>   , \r\"IDS0191_210310_RAW_cal__ref_\" ->   <|    \"ζ\" -> 0.025322625458   ,  \"τ1\" -> 0.023401812401   ,  \"τS\" -> 0.017347416709   ,  \"τN\" -> 0.002020498851   ,  \"τC\" -> 0.003594259467   ,  \"κ0\" -> 0.000000003970   ,  \"mm1\" -> 0.000074098080   ,  \"mm2\" -> 0.016429541452   ,  \"mm3\" -> 0.030350794367   ,  \"T\" -> 0.610000000000   ,  \"B\" -> 12.000000000000   ,  \"θ\" -> 90.000000000000   ,  \"Reoff\" -> 0.000000000000   ,  \"Imoff\" -> 0.000000000000    |>   , \r\"IDS0191_210310_RAW_cal__sam_\" ->   <|    \"ζ\" -> 0.020568815513   ,  \"τ1\" -> 0.023045965648   ,  \"τS\" -> 0.020791387386   ,  \"τN\" -> 0.002229171297   ,  \"τC\" -> 0.004427475438   ,  \"κ0\" -> 0.000000004398   ,  \"mm1\" -> 0.000074037290   ,  \"mm2\" -> 0.017820522459   ,  \"mm3\" -> 0.033072945644   ,  \"T\" -> 0.610000000000   ,  \"B\" -> 12.000000000000   ,  \"θ\" -> 90.000000000000   ,  \"Reoff\" -> 0.000000000000   ,  \"Imoff\" -> 0.000000000000    |>   , \r\"IDS0192_210310_RAW_cal__ref_\" ->   <|    \"ζ\" -> 0.022100596026   ,  \"τ1\" -> 0.020519097823   ,  \"τS\" -> 0.015555141042   ,  \"τN\" -> 0.000889956832   ,  \"τC\" -> 0.004354791503   ,  \"κ0\" -> 0.000000005560   ,  \"mm1\" -> 0.000074184851   ,  \"mm2\" -> 0.016476573734   ,  \"mm3\" -> 0.025131675080   ,  \"T\" -> 0.810000000000   ,  \"B\" -> 12.000000000000   ,  \"θ\" -> 90.000000000000   ,  \"Reoff\" -> 0.000000000000   ,  \"Imoff\" -> 0.000000000000    |>   , \r\"IDS0192_210310_RAW_cal__sam_\" ->   <|    \"ζ\" -> 0.016548170999   ,  \"τ1\" -> 0.020108887890   ,  \"τS\" -> 0.018558394948   ,  \"τN\" -> 0.001160732495   ,  \"τC\" -> 0.004746126241   ,  \"κ0\" -> 0.000000005882   ,  \"mm1\" -> 0.000061890920   ,  \"mm2\" -> 0.017029753868   ,  \"mm3\" -> 0.027808812278   ,  \"T\" -> 0.810000000000   ,  \"B\" -> 12.000000000000   ,  \"θ\" -> 90.000000000000   ,  \"Reoff\" -> 0.000000000000   ,  \"Imoff\" -> 0.000000000000    |>   , \r\"IDS0193_210310_RAW_cal__ref_\" ->   <|    \"ζ\" -> 0.020969814378   ,  \"τ1\" -> 0.020016820130   ,  \"τS\" -> 0.013372894745   ,  \"τN\" -> 0.000454586591   ,  \"τC\" -> 0.005292751338   ,  \"κ0\" -> 0.000000007771   ,  \"mm1\" -> 0.000078663474   ,  \"mm2\" -> 0.016609276996   ,  \"mm3\" -> 0.022739072051   ,  \"T\" -> 1.100000000000   ,  \"B\" -> 12.000000000000   ,  \"θ\" -> 90.000000000000   ,  \"Reoff\" -> 0.000000000000   ,  \"Imoff\" -> 0.000000000000    |>   , \r\"IDS0193_210310_RAW_cal__sam_\" ->   <|    \"ζ\" -> 0.014495870556   ,  \"τ1\" -> 0.019990087457   ,  \"τS\" -> 0.016832201384   ,  \"τN\" -> 0.000455517238   ,  \"τC\" -> 0.005555782498   ,  \"κ0\" -> 0.000000008420   ,  \"mm1\" -> 0.000060055560   ,  \"mm2\" -> 0.018114231010   ,  \"mm3\" -> 0.024909902538   ,  \"T\" -> 1.100000000000   ,  \"B\" -> 12.000000000000   ,  \"θ\" -> 90.000000000000   ,  \"Reoff\" -> 0.000000000000   ,  \"Imoff\" -> 0.000000000000    |>   , \r\"IDS0194_210310_RAW_cal__ref_\" ->   <|    \"ζ\" -> 0.020900896759   ,  \"τ1\" -> 0.018288874472   ,  \"τS\" -> 0.009095511262   ,  \"τN\" -> 0.000107884456   ,  \"τC\" -> 0.006896232004   ,  \"κ0\" -> 0.000000013449   ,  \"mm1\" -> 0.000081424831   ,  \"mm2\" -> 0.015492573296   ,  \"mm3\" -> 0.019006863291   ,  \"T\" -> 1.800000000000   ,  \"B\" -> 12.000000000000   ,  \"θ\" -> 90.000000000000   ,  \"Reoff\" -> 0.000000000000   ,  \"Imoff\" -> 0.000000000000    |>   , \r\"IDS0194_210310_RAW_cal__sam_\" ->   <|    \"ζ\" -> 0.014043763709   ,  \"τ1\" -> 0.018292068543   ,  \"τS\" -> 0.011311396743   ,  \"τN\" -> 0.000128802259   ,  \"τC\" -> 0.008087849636   ,  \"κ0\" -> 0.000000014258   ,  \"mm1\" -> 0.000065912054   ,  \"mm2\" -> 0.017276417784   ,  \"mm3\" -> 0.020638450794   ,  \"T\" -> 1.800000000000   ,  \"B\" -> 12.000000000000   ,  \"θ\" -> 90.000000000000   ,  \"Reoff\" -> 0.000000000000   ,  \"Imoff\" -> 0.000000000000    |>   , \r\"IDS0195_210310_RAW_cal__ref_\" ->   <|    \"ζ\" -> 0.019765118173   ,  \"τ1\" -> 0.018324978618   ,  \"τS\" -> 0.006054329354   ,  \"τN\" -> 0.000028420666   ,  \"τC\" -> 0.006398306925   ,  \"κ0\" -> 0.000000023958   ,  \"mm1\" -> 0.000061197185   ,  \"mm2\" -> 0.012449996348   ,  \"mm3\" -> 0.018415068303   ,  \"T\" -> 3.000000000000   ,  \"B\" -> 12.000000000000   ,  \"θ\" -> 90.000000000000   ,  \"Reoff\" -> 0.000000000000   ,  \"Imoff\" -> 0.000000000000    |>   , \r\"IDS0195_210310_RAW_cal__sam_\" ->   <|    \"ζ\" -> 0.016187684631   ,  \"τ1\" -> 0.018325345271   ,  \"τS\" -> 0.007510087776   ,  \"τN\" -> 0.000028419157   ,  \"τC\" -> 0.008115463080   ,  \"κ0\" -> 0.000000024747   ,  \"mm1\" -> 0.000062903858   ,  \"mm2\" -> 0.015524812312   ,  \"mm3\" -> 0.018513630087   ,  \"T\" -> 3.000000000000   ,  \"B\" -> 12.000000000000   ,  \"θ\" -> 90.000000000000   ,  \"Reoff\" -> 0.000000000000   ,  \"Imoff\" -> 0.000000000000    |>   , \r\"IDS0196_210310_RAW_cal__ref_\" ->   <|    \"ζ\" -> 0.030164668817   ,  \"τ1\" -> 0.012822215558   ,  \"τS\" -> 0.004108197943   ,  \"τN\" -> 0.000006999504   ,  \"τC\" -> 0.004420975765   ,  \"κ0\" -> 0.000000058872   ,  \"mm1\" -> 0.000063783415   ,  \"mm2\" -> 0.008574867378   ,  \"mm3\" -> 0.012843871546   ,  \"T\" -> 5.700000000000   ,  \"B\" -> 12.000000000000   ,  \"θ\" -> 90.000000000000   ,  \"Reoff\" -> 0.000000000000   ,  \"Imoff\" -> 0.000000000000    |>   , \r\"IDS0196_210310_RAW_cal__sam_\" ->   <|    \"ζ\" -> 0.027897403691   ,  \"τ1\" -> 0.014639690770   ,  \"τS\" -> 0.004105291179   ,  \"τN\" -> 0.000006999171   ,  \"τC\" -> 0.007414449545   ,  \"κ0\" -> 0.000000059701   ,  \"mm1\" -> 0.000073450671   ,  \"mm2\" -> 0.011534391407   ,  \"mm3\" -> 0.014673310811   ,  \"T\" -> 5.700000000000   ,  \"B\" -> 12.000000000000   ,  \"θ\" -> 90.000000000000   ,  \"Reoff\" -> 0.000000000000   ,  \"Imoff\" -> 0.000000000000    |>   , \r\"IDS0208_210310_RAW_cal__ref_\" ->   <|    \"ζ\" -> 0.000000000000   ,  \"τ1\" -> 0.000000000000   ,  \"τS\" -> 0.000000000000   ,  \"τN\" -> 0.000000000000   ,  \"τC\" -> 0.000000000000   ,  \"κ0\" -> 0.000000000000   ,  \"mm1\" -> 0.000000000000   ,  \"mm2\" -> 0.000000000000   ,  \"mm3\" -> 0.000000000000   ,  \"T\" -> 0.197000000000   ,  \"B\" -> 0.000000000000   ,  \"θ\" -> 0.000000000000   ,  \"Reoff\" -> 0.000000000000   ,  \"Imoff\" -> 0.000000000000    |>   , \r\"IDS0208_210310_RAW_cal__sam_\" ->   <|    \"ζ\" -> 0.000000000000   ,  \"τ1\" -> 0.000000000000   ,  \"τS\" -> 0.000000000000   ,  \"τN\" -> 0.000000000000   ,  \"τC\" -> 0.000000000000   ,  \"κ0\" -> 0.000000000000   ,  \"mm1\" -> 0.000000000000   ,  \"mm2\" -> 0.000000000000   ,  \"mm3\" -> 0.000000000000   ,  \"T\" -> 0.197000000000   ,  \"B\" -> 0.000000000000   ,  \"θ\" -> 0.000000000000   ,  \"Reoff\" -> 0.000000000000   ,  \"Imoff\" -> 0.000000000000    |>   , \r\"IDS0209_210310_RAW_cal__ref_\" ->   <|    \"ζ\" -> 0.163571654798   ,  \"τ1\" -> 0.020520714675   ,  \"τS\" -> 0.073117323271   ,  \"τN\" -> 0.020627224399   ,  \"τC\" -> 0.001336341391   ,  \"κ0\" -> 0.000000001061   ,  \"mm1\" -> 0.000185345173   ,  \"mm2\" -> 0.015331340913   ,  \"mm3\" -> 0.115418868440   ,  \"T\" -> 0.197000000000   ,  \"B\" -> 0.000000000000   ,  \"θ\" -> 0.000000000000   ,  \"Reoff\" -> 0.000000000000   ,  \"Imoff\" -> 0.000000000000    |>   , \r\"IDS0209_210310_RAW_cal__sam_\" ->   <|    \"ζ\" -> 0.132901556203   ,  \"τ1\" -> 0.022795175616   ,  \"τS\" -> 0.082481385864   ,  \"τN\" -> 0.041432545456   ,  \"τC\" -> 0.001408424074   ,  \"κ0\" -> 0.000000001182   ,  \"mm1\" -> 0.000163042447   ,  \"mm2\" -> 0.014386869823   ,  \"mm3\" -> 0.150035973048   ,  \"T\" -> 0.197000000000   ,  \"B\" -> 0.000000000000   ,  \"θ\" -> 0.000000000000   ,  \"Reoff\" -> 0.000000000000   ,  \"Imoff\" -> 0.000000000000    |>   , \r\"IDS0210_210310_RAW_cal__ref_\" ->   <|    \"ζ\" -> 0.000000000000   ,  \"τ1\" -> 0.000000000000   ,  \"τS\" -> 0.000000000000   ,  \"τN\" -> 0.000000000000   ,  \"τC\" -> 0.000000000000   ,  \"κ0\" -> 0.000000000000   ,  \"mm1\" -> 0.000000000000   ,  \"mm2\" -> 0.000000000000   ,  \"mm3\" -> 0.000000000000   ,  \"T\" -> 0.148000000000   ,  \"B\" -> 6.000000000000   ,  \"θ\" -> 0.000000000000   ,  \"Reoff\" -> 0.000000000000   ,  \"Imoff\" -> 0.000000000000    |>   , \r\"IDS0210_210310_RAW_cal__sam_\" ->   <|    \"ζ\" -> 0.000000000000   ,  \"τ1\" -> 0.000000000000   ,  \"τS\" -> 0.000000000000   ,  \"τN\" -> 0.000000000000   ,  \"τC\" -> 0.000000000000   ,  \"κ0\" -> 0.000000000000   ,  \"mm1\" -> 0.000000000000   ,  \"mm2\" -> 0.000000000000   ,  \"mm3\" -> 0.000000000000   ,  \"T\" -> 0.148000000000   ,  \"B\" -> 6.000000000000   ,  \"θ\" -> 0.000000000000   ,  \"Reoff\" -> 0.000000000000   ,  \"Imoff\" -> 0.000000000000    |>   , \r\"IDS0211_210310_RAW_cal__ref_\" ->   <|    \"ζ\" -> 0.160882265826   ,  \"τ1\" -> 0.034919932965   ,  \"τS\" -> 0.043973777096   ,  \"τN\" -> 0.047289018614   ,  \"τC\" -> 0.001339652100   ,  \"κ0\" -> 0.000000001069   ,  \"mm1\" -> 0.000181515969   ,  \"mm2\" -> 0.014272071349   ,  \"mm3\" -> 0.127751358817   ,  \"T\" -> 0.197000000000   ,  \"B\" -> 9.000000000000   ,  \"θ\" -> 0.000000000000   ,  \"Reoff\" -> 0.000000000000   ,  \"Imoff\" -> 0.000000000000    |>   , \r\"IDS0211_210310_RAW_cal__sam_\" ->   <|    \"ζ\" -> 0.132534999612   ,  \"τ1\" -> 0.042581417401   ,  \"τS\" -> 0.054103824371   ,  \"τN\" -> 0.072163013930   ,  \"τC\" -> 0.001421040158   ,  \"κ0\" -> 0.000000001190   ,  \"mm1\" -> 0.000162934689   ,  \"mm2\" -> 0.015546305497   ,  \"mm3\" -> 0.171294831040   ,  \"T\" -> 0.197000000000   ,  \"B\" -> 9.000000000000   ,  \"θ\" -> 0.000000000000   ,  \"Reoff\" -> 0.000000000000   ,  \"Imoff\" -> 0.000000000000    |>   , \r\"IDS0212_210310_RAW_cal__ref_\" ->   <|    \"ζ\" -> 0.154351103049   ,  \"τ1\" -> 0.051844552801   ,  \"τS\" -> 0.034651211615   ,  \"τN\" -> 0.065884588100   ,  \"τC\" -> 0.001166375427   ,  \"κ0\" -> 0.000000001084   ,  \"mm1\" -> 0.000152080810   ,  \"mm2\" -> 0.013701664106   ,  \"mm3\" -> 0.155210794609   ,  \"T\" -> 0.197000000000   ,  \"B\" -> 11.000000000000   ,  \"θ\" -> 0.000000000000   ,  \"Reoff\" -> 0.000000000000   ,  \"Imoff\" -> 0.000000000000    |>   , \r\"IDS0212_210310_RAW_cal__sam_\" ->   <|    \"ζ\" -> 0.124414912597   ,  \"τ1\" -> 0.052685716706   ,  \"τS\" -> 0.041788480794   ,  \"τN\" -> 0.092820346766   ,  \"τC\" -> 0.001183564004   ,  \"κ0\" -> 0.000000001217   ,  \"mm1\" -> 0.000128067207   ,  \"mm2\" -> 0.013191279693   ,  \"mm3\" -> 0.191906106886   ,  \"T\" -> 0.197000000000   ,  \"B\" -> 11.000000000000   ,  \"θ\" -> 0.000000000000   ,  \"Reoff\" -> 0.000000000000   ,  \"Imoff\" -> 0.000000000000    |>   , \r\"IDS0213_210310_RAW_cal__ref_\" ->   <|    \"ζ\" -> 0.158514180755   ,  \"τ1\" -> 0.046388884826   ,  \"τS\" -> 0.038847986012   ,  \"τN\" -> 0.058494864948   ,  \"τC\" -> 0.001325817289   ,  \"κ0\" -> 0.000000001072   ,  \"mm1\" -> 0.000176864175   ,  \"mm2\" -> 0.014706895751   ,  \"mm3\" -> 0.145604015421   ,  \"T\" -> 0.197000000000   ,  \"B\" -> 10.000000000000   ,  \"θ\" -> 0.000000000000   ,  \"Reoff\" -> 0.000000000000   ,  \"Imoff\" -> 0.000000000000    |>   , \r\"IDS0213_210310_RAW_cal__sam_\" ->   <|    \"ζ\" -> 0.130083148284   ,  \"τ1\" -> 0.046211117525   ,  \"τS\" -> 0.046173592526   ,  \"τN\" -> 0.081942172735   ,  \"τC\" -> 0.001380184863   ,  \"κ0\" -> 0.000000001209   ,  \"mm1\" -> 0.000155206642   ,  \"mm2\" -> 0.013836953800   ,  \"mm3\" -> 0.178380609297   ,  \"T\" -> 0.197000000000   ,  \"B\" -> 10.000000000000   ,  \"θ\" -> 0.000000000000   ,  \"Reoff\" -> 0.000000000000   ,  \"Imoff\" -> 0.000000000000    |>   , \r\"IDS0214_210310_RAW_cal__ref_\" ->   <|    \"ζ\" -> 0.154362032240   ,  \"τ1\" -> 0.030258273194   ,  \"τS\" -> 0.049523350330   ,  \"τN\" -> 0.040015703513   ,  \"τC\" -> 0.001328953616   ,  \"κ0\" -> 0.000000001075   ,  \"mm1\" -> 0.000174173720   ,  \"mm2\" -> 0.014698349376   ,  \"mm3\" -> 0.120075187874   ,  \"T\" -> 0.197000000000   ,  \"B\" -> 8.000000000000   ,  \"θ\" -> 0.000000000000   ,  \"Reoff\" -> 0.000000000000   ,  \"Imoff\" -> 0.000000000000    |>   , \r\"IDS0214_210310_RAW_cal__sam_\" ->   <|    \"ζ\" -> 0.126440702434   ,  \"τ1\" -> 0.034118036572   ,  \"τS\" -> 0.060921114440   ,  \"τN\" -> 0.059832148427   ,  \"τC\" -> 0.001404471084   ,  \"κ0\" -> 0.000000001199   ,  \"mm1\" -> 0.000154817132   ,  \"mm2\" -> 0.015271462818   ,  \"mm3\" -> 0.156117617951   ,  \"T\" -> 0.197000000000   ,  \"B\" -> 8.000000000000   ,  \"θ\" -> 0.000000000000   ,  \"Reoff\" -> 0.000000000000   ,  \"Imoff\" -> 0.000000000000    |>   , \r\"IDS0215_210310_RAW_cal__ref_\" ->   <|    \"ζ\" -> 0.162645417184   ,  \"τ1\" -> 0.023693851446   ,  \"τS\" -> 0.062400062170   ,  \"τN\" -> 0.026326088223   ,  \"τC\" -> 0.001322053294   ,  \"κ0\" -> 0.000000001070   ,  \"mm1\" -> 0.000182075033   ,  \"mm2\" -> 0.015525359924   ,  \"mm3\" -> 0.112465521923   ,  \"T\" -> 0.197000000000   ,  \"B\" -> 7.000000000000   ,  \"θ\" -> 0.000000000000   ,  \"Reoff\" -> 0.000000000000   ,  \"Imoff\" -> 0.000000000000    |>   , \r\"IDS0215_210310_RAW_cal__sam_\" ->   <|    \"ζ\" -> 0.131383255045   ,  \"τ1\" -> 0.026827335842   ,  \"τS\" -> 0.071725959535   ,  \"τN\" -> 0.047510049318   ,  \"τC\" -> 0.001407613780   ,  \"κ0\" -> 0.000000001187   ,  \"mm1\" -> 0.000160977956   ,  \"mm2\" -> 0.014932130994   ,  \"mm3\" -> 0.148043464486   ,  \"T\" -> 0.197000000000   ,  \"B\" -> 7.000000000000   ,  \"θ\" -> 0.000000000000   ,  \"Reoff\" -> 0.000000000000   ,  \"Imoff\" -> 0.000000000000    |>   , \r\"IDS0216_210310_RAW_cal__ref_\" ->   <|    \"ζ\" -> 0.149904026692   ,  \"τ1\" -> 0.020347243982   ,  \"τS\" -> 0.075273674904   ,  \"τN\" -> 0.020640082408   ,  \"τC\" -> 0.001432916876   ,  \"κ0\" -> 0.000000001050   ,  \"mm1\" -> 0.000184134986   ,  \"mm2\" -> 0.015328528282   ,  \"mm3\" -> 0.116559113338   ,  \"T\" -> 0.197000000000   ,  \"B\" -> 5.000000000000   ,  \"θ\" -> 0.000000000000   ,  \"Reoff\" -> 0.000000000000   ,  \"Imoff\" -> 0.000000000000    |>   , \r\"IDS0216_210310_RAW_cal__sam_\" ->   <|    \"ζ\" -> 0.125455081262   ,  \"τ1\" -> 0.021777951907   ,  \"τS\" -> 0.089086097551   ,  \"τN\" -> 0.033580911935   ,  \"τC\" -> 0.001437991682   ,  \"κ0\" -> 0.000000001167   ,  \"mm1\" -> 0.000158268021   ,  \"mm2\" -> 0.015150793318   ,  \"mm3\" -> 0.145963091379   ,  \"T\" -> 0.197000000000   ,  \"B\" -> 5.000000000000   ,  \"θ\" -> 0.000000000000   ,  \"Reoff\" -> 0.000000000000   ,  \"Imoff\" -> 0.000000000000    |>   , \r\"IDS0217_210310_RAW_cal__ref_\" ->   <|    \"ζ\" -> 0.121305227705   ,  \"τ1\" -> 0.032098202143   ,  \"τS\" -> 0.011865067519   ,  \"τN\" -> 0.005878702730   ,  \"τC\" -> 0.002147559783   ,  \"κ0\" -> 0.000000001032   ,  \"mm1\" -> 0.000202614262   ,  \"mm2\" -> 0.011552455211   ,  \"mm3\" -> 0.042386874792   ,  \"T\" -> 0.197000000000   ,  \"B\" -> 0.000000000000   ,  \"θ\" -> 0.000000000000   ,  \"Reoff\" -> 0.000000000000   ,  \"Imoff\" -> 0.000000000000    |>   , \r\"IDS0217_210310_RAW_cal__sam_\" ->   <|    \"ζ\" -> 0.101804363109   ,  \"τ1\" -> 0.031947692776   ,  \"τS\" -> 0.014125667853   ,  \"τN\" -> 0.006009042128   ,  \"τC\" -> 0.002323789932   ,  \"κ0\" -> 0.000000001168   ,  \"mm1\" -> 0.000188754224   ,  \"mm2\" -> 0.013103876414   ,  \"mm3\" -> 0.043163363377   ,  \"T\" -> 0.197000000000   ,  \"B\" -> 0.000000000000   ,  \"θ\" -> 0.000000000000   ,  \"Reoff\" -> 0.000000000000   ,  \"Imoff\" -> 0.000000000000    |>   , \r\"IDS0218_210310_RAW_cal__ref_\" ->   <|    \"ζ\" -> 0.000000000000   ,  \"τ1\" -> 0.000000000000   ,  \"τS\" -> 0.000000000000   ,  \"τN\" -> 0.000000000000   ,  \"τC\" -> 0.000000000000   ,  \"κ0\" -> 0.000000000000   ,  \"mm1\" -> 0.000000000000   ,  \"mm2\" -> 0.000000000000   ,  \"mm3\" -> 0.000000000000   ,  \"T\" -> 1.550000000000   ,  \"B\" -> 0.000000000000   ,  \"θ\" -> 0.000000000000   ,  \"Reoff\" -> 0.000000000000   ,  \"Imoff\" -> 0.000000000000    |>   , \r\"IDS0218_210310_RAW_cal__sam_\" ->   <|    \"ζ\" -> 0.000000000000   ,  \"τ1\" -> 0.000000000000   ,  \"τS\" -> 0.000000000000   ,  \"τN\" -> 0.000000000000   ,  \"τC\" -> 0.000000000000   ,  \"κ0\" -> 0.000000000000   ,  \"mm1\" -> 0.000000000000   ,  \"mm2\" -> 0.000000000000   ,  \"mm3\" -> 0.000000000000   ,  \"T\" -> 1.550000000000   ,  \"B\" -> 0.000000000000   ,  \"θ\" -> 0.000000000000   ,  \"Reoff\" -> 0.000000000000   ,  \"Imoff\" -> 0.000000000000    |>   , \r\"IDS0219_210310_RAW_cal__ref_\" ->   <|    \"ζ\" -> 0.000000000000   ,  \"τ1\" -> 0.000000000000   ,  \"τS\" -> 0.000000000000   ,  \"τN\" -> 0.000000000000   ,  \"τC\" -> 0.000000000000   ,  \"κ0\" -> 0.000000000000   ,  \"mm1\" -> 0.000000000000   ,  \"mm2\" -> 0.000000000000   ,  \"mm3\" -> 0.000000000000   ,  \"T\" -> 1.000000000000   ,  \"B\" -> 0.000000000000   ,  \"θ\" -> 0.000000000000   ,  \"Reoff\" -> 0.000000000000   ,  \"Imoff\" -> 0.000000000000    |>   , \r\"IDS0219_210310_RAW_cal__sam_\" ->   <|    \"ζ\" -> 0.000000000000   ,  \"τ1\" -> 0.000000000000   ,  \"τS\" -> 0.000000000000   ,  \"τN\" -> 0.000000000000   ,  \"τC\" -> 0.000000000000   ,  \"κ0\" -> 0.000000000000   ,  \"mm1\" -> 0.000000000000   ,  \"mm2\" -> 0.000000000000   ,  \"mm3\" -> 0.000000000000   ,  \"T\" -> 1.000000000000   ,  \"B\" -> 0.000000000000  
